vi "GetType.vi"(8 "error in (no error)":errorcluster, 11 "Set Length Msg":refnum<class "Set Length Msg.lvclass">) -> (0 "error out":errorcluster, 2 "Data Sample":variant, 3 "Set Length Msg":refnum<class "Set Length Msg.lvclass">)   [LabVIEW 2020, in "BNT_ULx.lvlib" / "Set Length Msg.lvclass"]
uses:
  Set Length Msg.lvclass
  Set Length Msg.lvclass/Set Length Msg.ctl
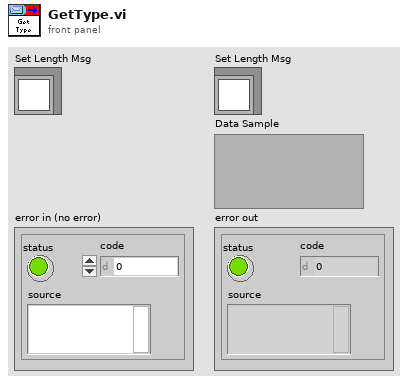
[diagram p1: front panel]
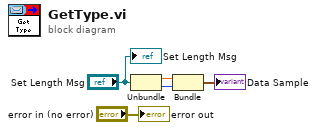
[diagram p0: block diagram]
diagram:
  n1 = Unbundle("Set Length Msg") -> (w2:dbl[unit], w1:i32)
  n2 = Bundle("PWM Length"=w2, "Line"=w1) -> (→"Data Sample":cluster{"PWM Length":dbl[unit], "Line":i32})  [unwired: 1 in]
  "error out" <- "error in (no error)"
  "Set Length Msg" <- "Set Length Msg"
